vi "GF_ArmAgilentSingle.vi"(0 "Agilent Control In":T1={"Trig?"=FALSE, "VISA session"="Agilent6034", "Setup to Load"="2", "Timeout (ms)"=40000, "Desired Samp"=enum."1000", "Captured Samp"=11, "Desired Channels"=[{"Chan Index"=enum."Channel1", "Name"="Chan1Test", "Samples"=0}, {"Chan Index"=enum."Channel2", "Name"="Chan2Test", "Samples"=0}, {"Chan Index"=enum."Channel3", "Name"="Chan3Test", "Samples"=0}, {"Chan Index"=enum."Channel4", "Name"="Chan4Test", "Samples"=0}]}) -> (1 "Agilent Control Out":T1={"Trig?"=FALSE, "VISA session"="Agilent6034", "Setup to Load"="2", "Timeout (ms)"=40000, "Desired Samp"=enum."1000", "Captured Samp"=11, "Desired Channels"=[{"Chan Index"=enum."Channel1", "Name"="Chan1Test", "Samples"=0}, {"Chan Index"=enum."Channel2", "Name"="Chan2Test", "Samples"=0}, {"Chan Index"=enum."Channel3", "Name"="Chan3Test", "Samples"=0}, {"Chan Index"=enum."Channel4", "Name"="Chan4Test", "Samples"=0}]}, 2 "Agilent Present":bool=TRUE, 3 "Agilent Setup Error":errorcluster)   [LabVIEW 2020]
uses:
  AgilentControl.ctl
  Channel Config.ctl
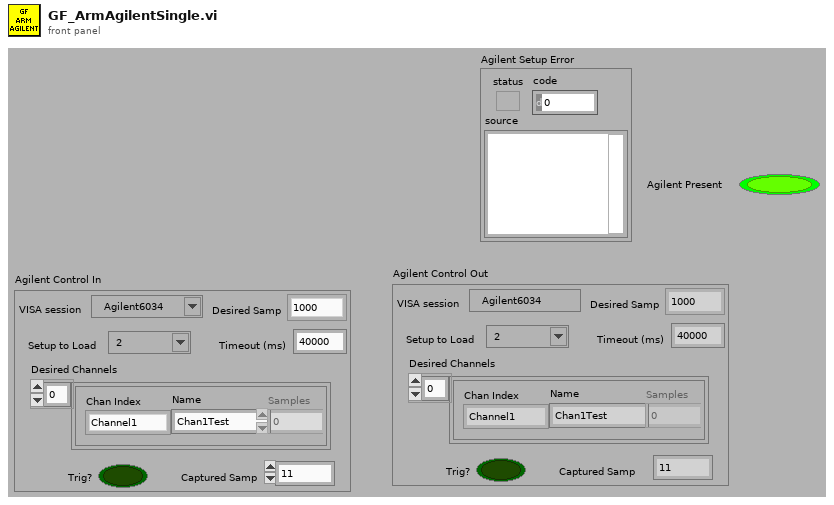
[diagram p1: front panel]
types:
  T1 = typedef "AgilentControl.ctl" = cluster{"Trig?":bool, "VISA session":refnum<visa-resource-name>, "Setup to Load":string, "Timeout (ms)":u32, "Desired Samp":enum32{"100", "250", "500", "1000", "2000", "5000", "10000", "20000", "50000", "100000", "200000", "500000", "1000000", "2000000", "4000000", "8000000"}, "Captured Samp":i32, "Desired Channels":T2[]}
  T2 = typedef "Channel Config.ctl" = cluster{"Chan Index":enum16{"Channel1", "Channel2", "Channel3", "Channel4", "MATH"}, "Name":string, "Samples":i32}
  T3 = enum32{"100", "250", "500", "1000", "2000", "5000", "10000", "20000", "50000", "100000", "200000", "500000", "1000000", "2000000", "4000000", "8000000"}
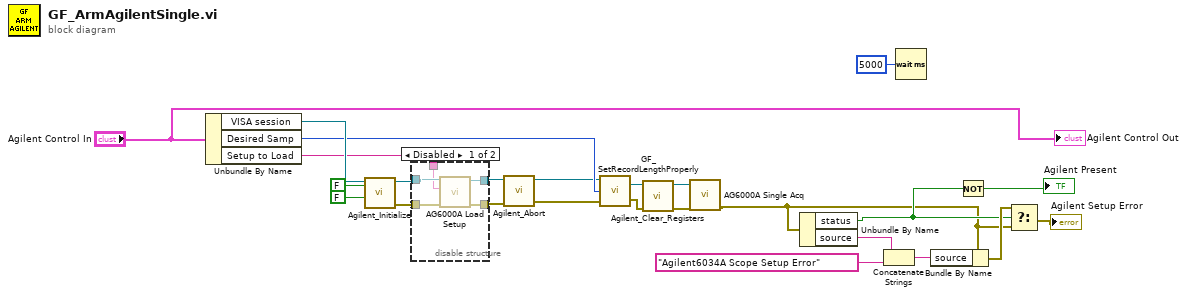
[diagram p0: block diagram]
diagram:
  n1 = Unbundle By Name("Agilent Control In") -> ("VISA session"=w22:refnum<visa-resource-name>, "Desired Samp"=w21:T3, "Setup to Load"=w20:string)
  n2 = call "Agilent_Initialize.vi"("Reset? (T: Yes)"=FALSE, "ID Query? (T: Yes)"=FALSE, "VISA resource name"=w22) -> ("error out"=w24:errorcluster, "VISA resource name out"=w25:refnum<visa-resource-name>)  [unwired: 7 in]
  n3 = disable-structure shown="Disabled" {
    disable-tunnel: [w30 w31] -> w11
    disable-tunnel: [w29 w32] -> w12
    disable-tunnel: w25 -> [w28 w31]
    disable-tunnel: w24 -> [w27 w32]
    disable-tunnel: w20 -> [w26 _]
    frame Disabled {
      n4 = call "AG6000A Load Setup.vi"("error in (no error)"=w27, "Setup to Load"=w26, "VISA session"=w28) -> ("error out"=w29:errorcluster, "dup VISA session"=w30:refnum<visa-resource-name>)  [unwired: 7 in]
    }
    frame Enabled {
    }
  }
  n5 = call "Agilent_Abort.vi"("error in (no error)"=w12, "VISA resource name"=w11) -> ("error out"=w1:errorcluster, "VISA resource name out"=w2:refnum<visa-resource-name>)  [unwired: 8 in]
  n6 = call "GF_SetRecordLengthProperly.vi"("error in (no error)"=w1, "Num Samples"=w21, "VISA resource name"=w2) -> ("error out"=w7:errorcluster, "VISA resource name out"=w8:refnum<visa-resource-name>)
  n7 = call "Agilent_Clear_Registers.vi"("error in (no error)"=w7, "VISA session"=w8) -> ("error out"=w5:errorcluster, "dup VISA session"=w6:refnum<visa-resource-name>)  [unwired: 8 in]
  n8 = call "AG6000A Single Acq.vi"("error in (no error)"=w5, "VISA session"=w6) -> ("error out"=w4:errorcluster)  [unwired: 8 in, 1 out]
  n9 = Unbundle By Name(w4) -> ("status"=w15:bool, "source"=w19:string)
  n10 = Concatenate Strings(w19, "Agilent6034A Scope Setup Error") -> (w18:string)
  n11 = Wait (ms)(milliseconds to wait=u32 5000) -> ()  [unwired: 1 out]
  n12 = Bundle By Name(cluster=w4, "source"=w18) -> (w16:errorcluster)
  n13 = Not(x=w15) -> (.not. x?=→"Agilent Present":bool)
  n14 = Select(t=w16, s=w15, f=w4) -> (s? t:f=→"Agilent Setup Error":errorcluster)
  "Agilent Control Out" <- "Agilent Control In"
